vi "Generate Unique Header.vi"(8 "error in":errorcluster, 11 "Data in":refnum<class "Data.lvclass">) -> (0 "error out":errorcluster, 2 "Header":string[](array[string]), 3 "Data out":refnum<class "Data.lvclass">)   [LabVIEW 2016, in "Base Data Class.lvlib" / "Data.lvclass"]
uses:
  Data.lvclass
  Data.lvclass/Data.ctl
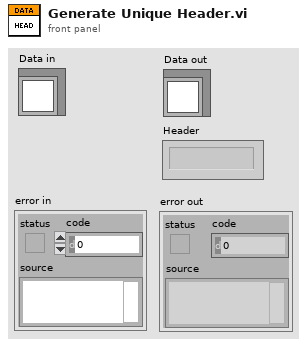
[diagram p1: front panel]
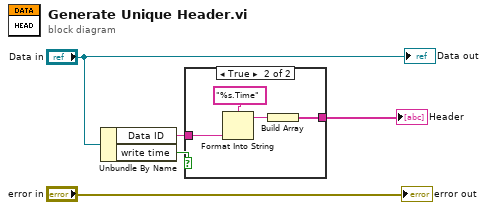
[diagram p0: block diagram]
diagram:
  n1 = Unbundle By Name("Data in") -> ("Data ID"=w2:string, "write time"=w1:bool)
  n2 = case shown="True" w1 {
    tunnel: [_ w9] -> w4
    tunnel: w2 -> [_ w6]
    frame False {
    }
    frame True {
      n3 = Format Into String(format string="%s.Time", w6) -> (resulting string=w7:string)  [unwired: 2 in, 1 out]
      n4 = Build Array(w7) -> (w9:string[])
    }
  }
  "Header" <- w4
  "error out" <- "error in"
  "Data out" <- "Data in"
